vi "testArea.vi"   [LabVIEW 2019]
uses:
  <vilib>/addons/VCD Debug Tools/Examples/VCD Debug Tools Examples.lvlib
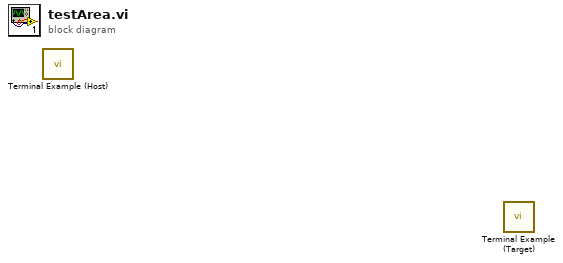
[diagram p0: block diagram]
diagram:
  n1 = call <vilib>:"Terminal Example (Host).vi"() -> ()  [unwired: 12 in]
  n2 = call <vilib>:"Terminal Example (Target).vi"() -> ()  [unwired: 12 in]
